vi "Get Time.vi"(0 "reference in":refnum<class "Timer.lvclass">, 5 "error in (no error)":errorcluster) -> (14 "reference out":refnum<class "Timer.lvclass">, 16 "Timer Time (min)":dbl, 17 "Timer Time (s)":dbl, 18 "Timer Time (ms)":u32, 19 "error out":errorcluster)   [LabVIEW 2017, in "Timer.lvclass"]
uses:
  Timer.lvclass
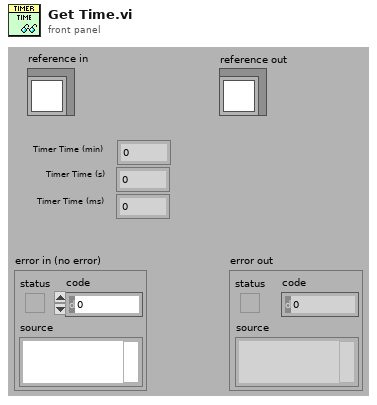
[diagram p1: front panel]
types:
  T1 = typedef "Timer.lvclass/ObjectAttributes.ctl" = cluster{"Timer is Timing":bool, "Timer Time (ms)":u32, "Timer VI Reference":refnum<vi>}
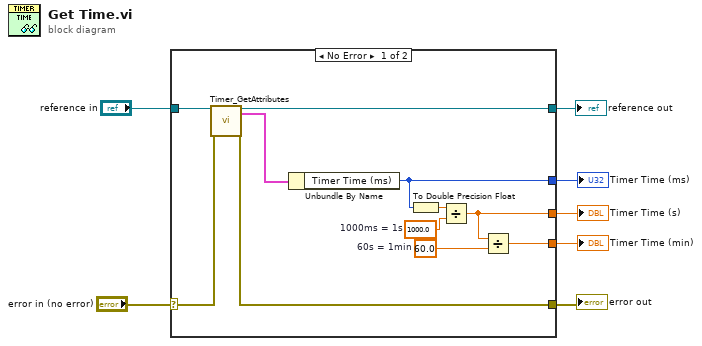
[diagram p0: block diagram]
diagram:
  n1 = case shown="No Error" "error in (no error)" {
    selector: "error in (no error)" -> [w18 w20]
    tunnel: [w16 w20] -> w6
    tunnel: [w14 w19] -> w4
    tunnel: "reference in" -> [w15 w19]
    tunnel: [w12 _] -> w3
    tunnel: [w11 _] -> w2
    tunnel: [w9 _] -> w1
    frame No Error {
      w8 = 60.0  # 60s = 1min
      w10 = 1000.0  # 1000ms = 1s
      n2 = call "Timer_GetAttributes.vi"("reference in"=w15, "error in (no error)"=w18) -> ("reference out"=w14:refnum<class "Timer.lvclass">, "Data"=w17:T1, "error out"=w16:errorcluster)  [unwired: 14 in, 1 out]
      n3 = Unbundle By Name(w17) -> ("Timer Time (ms)"=w12:u32)
      n4 = To Double Precision Float(number=w12) -> (double precision float=w13:dbl)
      n5 = Divide(x=w13, y=w10) -> (x/y=w11:dbl)
      n6 = Divide(x=w11, y=w8) -> (x/y=w9:dbl)
    }
    frame Error {
    }
  }
  "error out" <- w6
  "reference out" <- w4
  "Timer Time (ms)" <- w3
  "Timer Time (s)" <- w2
  "Timer Time (min)" <- w1
